vi "Save All Tables.vi"(2 "Error In":errorcluster, 3 "File Path":string, 4 "SaveOption(Temporary File)":T1) -> (0 "Error Out":errorcluster, 1 "Path":path)   [LabVIEW 2018]
uses:
  Type Defs/Save Options.ctl
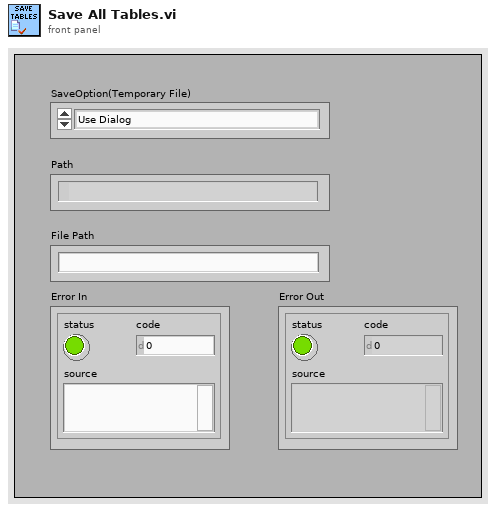
[diagram p1: front panel]
types:
  T1 = typedef "Save Options.ctl" = enum16{"Use Dialog", "Temporary File", "My Tables", "Full Path"}
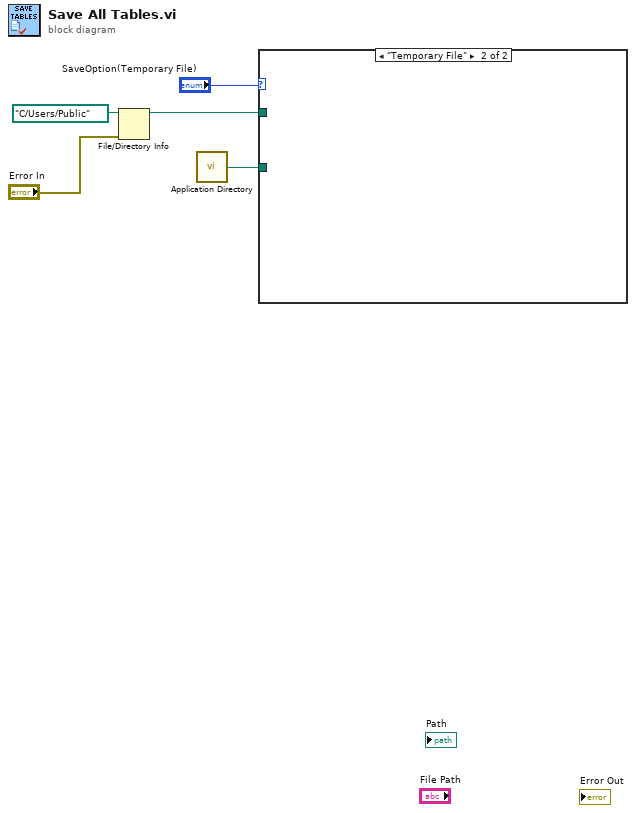
[diagram p0: block diagram]
diagram:
  n1 = File/Directory Info(path=path "C:/Users/Public" ("stripped path"), error in="Error In") -> (path out=w2:path)  [unwired: 6 out]
  n2 = call <vilib>:"Application Directory.vi"() -> ("Application Directory"=w1:path)
  n3 = case shown="\"Temporary File\"" "SaveOption(Temporary File)" {
    tunnel: w2 -> [_ _]
    tunnel: w1 -> [_ _]
    frame "Use Dialog", Default {
    }
    frame "Temporary File" {
    }
  }
